vi "数组初始化.vi"() -> ()   [LabVIEW 2018]
panel:
  out "数组":dbl[][](array[numeric])
  in  "列":i32
  in  "行":i32
  in  "元素":dbl
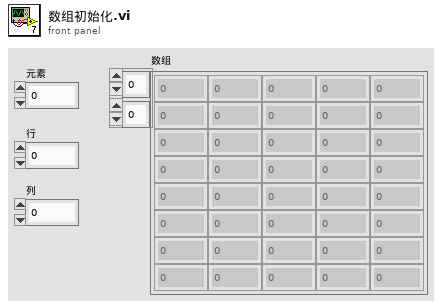
[diagram p1: front panel]
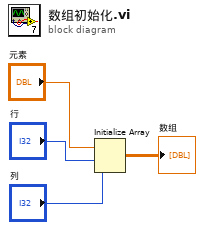
[diagram p0: block diagram]
diagram:
  n1 = Initialize Array("元素", "行", "列") -> (→"数组":dbl[][])
